vi "Phoenix.vi"() -> ()   [LabVIEW 2020]
uses:
  Vision_class/Old vision/SSL Detection Frame Simple Estimator Cameras VelCmd Folder/Core/AI Input.ctl
  Vision_class/Old vision/Controls/AI Robot.ctl
  Vision_class/Old vision/Controls/Functions Enum.ctl
  Vision_class/Old vision/Controls/AttackerStates.ctl
  Vision_class/Old vision/Controls/PathDests.ctl
  Vision_class/Old vision/Controls/PathDest.ctl
  Vision_class/Old vision/SSL Detection Frame Simple Estimator Cameras VelCmd Folder/Core/AI Ball.ctl
  Vision_class/Old vision/SSL Detection Frame Simple Estimator Cameras VelCmd Folder/Core/Field Size.ctl
  Vision_class/Old vision/SSL Detection Frame Simple Estimator Cameras VelCmd Folder/Core/AI Judge.ctl
  Communication_class/Paths/MessageAI_State Folder/Intel/Command Enum.ctl
  Vision_class/Old vision/SSL Detection Frame Simple Estimator Cameras VelCmd Folder/Util/Events/Events.ctl
  Vision_class/Old vision/Controls/Estimadores.ctl
  Vision_class/Old vision/Decode SSL and Refree Wrapper Package Folder/SSL Referee Game Status.ctl
  Vision_class/Old vision/Draw Field Folder/DrawTargets.ctl
  Vision_class/Old vision/Controls/SSL Field State.ctl
  Vision_class/Old vision/Controls/SSL Detection Frame.ctl
  Vision_class/Old vision/Controls/SSL Detection Robot.ctl
  <vilib>/Analysis/Matrix/Datatypes/RealMatrix.ctl
  Vision_class/Old vision/Controls/SSL Detection Ball.ctl
  Communication_class/Communication.lvclass
  Controls/ComUDP.ctl
  Controls/ComSerial.ctl
  Controls/ComSOS.ctl
  Controls/vision_control.ctl
  Team_class/KeeperPlay.ctl
  Team_class/OffensivePlay.ctl
  Referee_class/command_interpreted.ctl
  Robot_class/roles.ctl
  Robot_class/tactics.ctl
  Team_class/DefensivePlay.ctl
  Communication_class/Paths/grSim Packet Command UDP Test Folder/grSim/grSim RobotReplacement.ctl
  Communication_class/Paths/grSim Packet Command UDP Test Folder/grSim/grSim_BallReplacement.ctl
  Vision_class/Vision.lvclass
  Game_class/Game.lvclass
  Game_class/Game.lvclass/Game.ctl
  Parameters_class/Parameters.lvclass/Parameters.ctl
  Robot_class/Robot.lvclass
  Team_class/Team.lvclass/Team.ctl
  Events_class/Events.lvclass
  Referee_class/Referee.lvclass/Referee.ctl
  Robot_class/Robot.lvclass/Robot.ctl
  Game_class/Read KeeperTeam.vi
  Game_class/Write KeeperTeam.vi
  Game_class/Write Offensive ids.vi
  Game_class/Write Defensive ids.vi
  Game_class/Read Parameters.lvclass.vi
  Game_class/Write TestMode IDs.vi
  Game_class/Write TestMode.vi
  Game_class/Write Tests.vi
  Parameters_class/Write Area.vi
  Parameters_class/Write DistanceBehindAttacker.vi
  Parameters_class/Write DistanceInFrontOfAttacker.vi
  Parameters_class/Write DistanceStop.vi
  Parameters_class/Write DistanceToBallOut.vi
  Parameters_class/Write DistanceToGoAroundBall.vi
  Parameters_class/Write DistanceToGoAroundBallPass.vi
  Parameters_class/Write DistanceToKickingAngle.vi
  Parameters_class/Write Force++.vi
  Parameters_class/Write KickAngle.vi
  Parameters_class/Write KickEps.vi
  Parameters_class/Write KickForce.vi
  Parameters_class/Write KickRange.vi
  Parameters_class/Write MaxAcceleration.vi
  Parameters_class/Write MaxControlIncrement.vi
  Parameters_class/Write MaxDeceleration.vi
  Parameters_class/Write MaxOutputAngle.vi
  Parameters_class/Write MaxOutputXY.vi
  Parameters_class/Write MinDistToKick.vi
  Parameters_class/Write PassAngle.vi
  Parameters_class/Write Type of Marker.vi
  Parameters_class/Write AttackerFarback.vi
  Parameters_class/Write TouchDistance.vi
  Parameters_class/Write TimeoutDistanceInY.vi
  Parameters_class/Write TimeoutDistanceInX.vi
  Parameters_class/Write TimeoutDistanceBetweenRobots.vi
  Parameters_class/Write DistanceForPossession.vi
  Parameters_class/Write DistanceForaStillBall.vi
  Parameters_class/Write AngularToleranceForPossession.vi
  Parameters_class/Write AttakingOurselves.vi
  Parameters_class/Write Debug.vi
  Parameters_class/Write ChipKick activated.vi
  Parameters_class/Write Angle.vi
  Parameters_class/Write PID gains Vel.vi
  Parameters_class/Write PID gains Vel_desired.vi
  Parameters_class/Write PID gains Angle.vi
  Parameters_class/Write Number of Offesnive.vi
  Parameters_class/Write Shoot Out_.vi
  Parameters_class/Write DefenseAvoidArea.vi
  Parameters_class/Write InvertKick.vi
  Game_class/Write Parameters.lvclass.vi
  Game_class/Read DefensiveTeam.vi
  Team_class/Read RobotRef.vi
  Game_class/Read OffensiveTeam.vi
  Game_class/Read AllyRef.vi
  Team_class/Write RobotRef.vi
  Game_class/Write NavigationTeam.vi
  Game_class/Write EventsRef.vi
  Game_class/Write OffensiveTeam.vi
  Robot_class/Read id.vi
  Robot_class/Read role.vi
  Robot_class/Read tactic.vi
  Game_class/Read Referee.vi
  Team_class/Read DefensivePlay.vi
  Team_class/Read OffensivePlay.vi
  Team_class/Read KeeperPlay.vi
  Referee_class/Read command_interpreted.vi
  Game_class/Read EventsRef.vi
  Ally_class/Ally.lvclass
  Playbook_class/Playbook.lvclass
  Parameters_class/Parameters.lvclass
  Referee_class/Referee.lvclass
  Utilities_class/Utilities.lvclass
  <vilib>/Analysis/Matrix/NI_Matrix.lvlib
panel:
  out "FPS vision 2":dbl
  out "FPS Offensive 2":dbl
  in  "grSIM replacement":cluster{"robots":T1[], "ball":T2}
  in  "replace active":bool
  out "Vel estimativa":T3(graph)
  out "Vel cmd":T3(graph)
  in  "Debug":bool
  out "tempo udp":dbl
  in  "ball out":bool
  in  "ball velocity máx":dbl=20.0
  in  "PID gains Angle":cluster{"(Kc)":dbl, "(Ki)":dbl, "(Kd)":dbl}={"(Kc)"=5.0, "(Ki)"=0.1, "(Kd)"=-1.0}
  in  "PID gains Vel D":cluster{"(Kp)":dbl, "(Ki)":dbl, "(Kd)":dbl}={"(Kp)"=20.0, "(Ki)"=100.0, "(Kd)"=0.5}
  in  "ChipKick activated":bool
  out "error out":errorcluster
  in  "Draw Graphs":bool
  out "zoom":dbl
  in  "Test":bool
  in  "Tab Control":T4(tab)
  in  "Com UDP":T5={"UDP GrSim TX"=TRUE, "Address:"="127.0.0.1", "Port:"=20011}
  in  "Com Serial":T6={"Serial TX"=FALSE, "Porta:"="COM12"}
  in  "Com SOS":T7={"UDP SOS TX "=FALSE, "SOS Port: 2"=10025, "SOS Port: "=10021, "SOS Address:"="192.168.0.101"}
  in  "RefBox UDP RX":T8={"Local IP:"="", "Port"=10003, "Server IP:"="224.5.23.1"}
  out "RefBox RX":bool
  in  "Defense\n stretch":i32=2000
  in  "Defense\n width":i32=1000
  in  "Team":enum16{"Azul", "Amarelo"}(ring) caption="Enum"
  in  "Side":enum16{"Esquerdo", "Direito"}(ring) caption="Enum"
  in  "Goalie":string(combo)="0"
  in  "Command":string(combo)="Auto"
  in  "AttakingOurselves":bool
  out "SSL RX":bool
  in  "SSL UDP RX":T8={"Local IP:"="", "Port"=10020, "Server IP:"="224.5.23.2"}
  out "KeeperPlay":T9=enum."NormalGame"
  out "OffensivePlay":T10=enum."TestPlay"
  out "Keeper Team":cluster{"id":i32, "role":T11, "tactic":T12}[](array[cluster])
  out "Offensive Team":cluster{"id":i32, "role":T11, "tactic":T12}[](array[cluster])
  out "Defensive Team":cluster{"id":i32, "role":T11, "tactic":T12}[](array[cluster])
  out "DefensivePlay":T13=enum."Halt"
  in  "TestMode IDS":dbl[](array[numeric])
  out "SSL Referee Game Status":T14 {"Time" format="%<%.3X %x>T"; "Blue Timeout Remaining" format="%<%M:%S>t"; "Yellow Timeout Remaining" format="%<%M:%S>t"; "Time Left" format="%<%M:%S>t"}
  out "FPS Offensive":dbl
  out "FPS SetParameters":dbl
  out "FPS Com":dbl
  out "FPS Draw Field":dbl
  out "FPS Graph":dbl
  out "FPS referee":dbl
  out "FPS vision":dbl
  out "FPS Events":dbl
  out "FPS Mouse":dbl
  out "FPS Print Field":dbl
  in  "zigzag Points":cluster{"x":dbl, "y":dbl, "Angle":dbl}[](array[cluster])=[{"x"=-4300.0, "y"=-3000.0, "Angle"=0.0}, {"x"=-4300.0, "y"=3000.0, "Angle"=0.0}, {"x"=-100.0, "y"=3000.0, "Angle"=0.0}, {"x"=-4300.0, "y"=3000.0, "Angle"=0.0}]
  in  "TestMode":bool
  in  "Tests":enum16{"zigzag", "goto"}(ring)
  in  "Offensive ids":dbl[](array[numeric])
  in  "Defensive ids":dbl[](array[numeric])
  out "command_interpreted":T15=enum."Halt"
  out "FPS Navigation":dbl
  out "FPS Read UDP":dbl
  in  "id 3":dbl
  in  "id 2":dbl
  in  "id 1":dbl
  out "Robot":cluster{"Modulo":dbl, "Modulo":dbl}(graph)
  out "Robot":cluster{"Modulo":dbl, "Modulo":dbl}(graph)
  out "Robot":cluster{"Modulo":dbl, "Modulo":dbl}(graph)
  out "ball":dbl(graph)
  in  "AI Parameters":T16={"Defensive Marker"=enum."SecondMostDangerous", "TimeoutDistanceInX"=600.0, "TimeoutDistanceInY"=600.0, "DistanceForaStillBall"=0.0, "TouchDistance"=130.0, "AttackerFarback"=1500.0, "MinDistToKick"=150.0, "Type of Marker"=enum."BlockEnemyPass", "Type of Defense "=enum."Manmark", "PassAngle"=0.045, "KickRange"=60.0, "KickForce"=100.0, "KickEps"=0.05, "KickAngle"=0.09, "Force++"=5.0, "DistanceToKickingAngle"=150.0, "DistanceToBallOut"=600.0, "DistanceStop"=600.0, "DistanceBehindAttacker"=200.0, "Area"=enum."Square", "DistanceForPossession"=180.0, "DistanceToGoAroundBallPass"=0.0, "DistanceToGoAroundBall"=200.0, "DistanceInFrontOfAttacker"=200.0, "TimeoutDistanceBetweenRobots"=300.0, "MaxOutputAngle"=4.0, "MaxOutputXY"=1.0, "MaxDeceleration"=1.0, "MaxControlIncrement"=1.0, "MaxAcceleration"=4.0, "AngularToleranceForPossession"=0.3, "MaxVelBallToBeginDuelist"=0.5, "ZigZagAngle"=0.0, "PID gains Vel"={"(Kc)"=0.0, "(Ti, min)"=0.0, "(Td, min)"=0.0}, "Number of Offensive"=enum."Auto", "Shoot Out?"=FALSE, "DefenseAvoidArea"=FALSE, "InvertKick"=[]}
  in  "Id camera\ninf dir":dbl=2.0
  in  "Id camera\ninf esq":dbl
  in  "Id camera\nsup dir":dbl=3.0
  in  "Id camera\nsup esq":dbl=1.0
  in  "ignore left?":bool
  in  "ignore rigth?":bool
  in  "Estimador":T17=enum."Kalman"
  in  "Draw Targets?":T18={"Attacker"=TRUE, "Striker"=TRUE, "Goalie"=TRUE, "Defender"=TRUE, "kick"=TRUE, "Est Ball"=TRUE, "Est Robot"=FALSE, "Path S"=FALSE, "Path C"=FALSE, "Dngr.Enemy"=TRUE, "2nd Striker"=TRUE}
  in  "Draw Field":bool=TRUE
  in  "Communication in":refnum<class "Communication.lvclass">
  in  "Frame and Field Size out Ref":T19 {"Detection Frame Out"."robots_blue"."height" format="%+4.3f"; "Detection Frame Out"."robots_blue"."pixel_y" format="%+4.3f"; "Detection Frame Out"."robots_blue"."pixel_x" format="%+4.3f"; "Detection Frame Out"."robots_blue"."orientation" format="%+4.3f"; "Detection Frame Out"."robots_blue"."y" format="%+4.3f"; "Detection Frame Out"."robots_blue"."confidence" format="%4.3f"; "Detection Frame Out"."robots_blue"."x" format="%+4.3f"; "Detection Frame Out"."robots_yellow"."height" format="%+4.3f"; "Detection Frame Out"."robots_yellow"."pixel_y" format="%+4.3f"; "Detection Frame Out"."robots_yellow"."pixel_x" format="%+4.3f"; "Detection Frame Out"."robots_yellow"."orientation" format="%+4.3f"; "Detection Frame Out"."robots_yellow"."y" format="%+4.3f"; "Detection Frame Out"."robots_yellow"."confidence" format="%4.3f"; "Detection Frame Out"."robots_yellow"."x" format="%+4.3f"}
  out "2D Picture":picture
  in  "SSL Referee Game Status Ref":T14 {"Time" format="%<%.3X %x>T"; "Blue Timeout Remaining" format="%<%M:%S>t"; "Yellow Timeout Remaining" format="%<%M:%S>t"; "Time Left" format="%<%M:%S>t"}
  out "GUI Game Status":T14 {"Time" format="%<%.3X %x>T"; "Blue Timeout Remaining" format="%<%M:%S>t"; "Yellow Timeout Remaining" format="%<%M:%S>t"; "Time Left" format="%<%M:%S>t"}
  out "AI State":T24={"our_robots"=[], "enemy_robots"=[], "balls"=[], "geometry"={"line_width"=0, "field_length"=0, "field_width"=0, "boundary_width"=0, "referee_width"=0, "goal_width"=0, "goal_depth"=0, "goal_wall_width"=0, "center_circle_radius"=0, "defense_radius"=0, "defense_stretch"=0, "free_kick_from_defense_dist"=0, "penalty_spot_from_field_line_dist"=0, "penalty_line_from_spot_dist"=0}, "IA Judge"={"stage"="", "command"="", "our_goalie_id"=0.0, "enemy_goalie_id"=0.0, "command enum"=enum."Halt", "Time"=enum."Azul"}, "Received Timestamp"=timestamp(0 s since 1904-01-01), "Events"={"Touch"=FALSE, "Ball out"=FALSE, "id touch"=0.0, "Ball out of \nVision"=FALSE, "Ball inside \nGoalie area"=FALSE, "Robot not responding"=FALSE, "Robots responding status"=[1.0, 1.0, 1.0, 1.0, 1.0, 1.0], "Enemy Ball \nPossession"=FALSE, "Pass State"=FALSE, "id end of pass"=0.0, "Kick"=FALSE, "Id ini Possession"=0.0, "Ball Possesion"=FALSE, "Id Possesion"=0.0, "Direct Kick"=FALSE, "2nd Strk Ativo"=FALSE}}
  # "To execute Test and TestMode(zigzag)\nthe referee command must be Stop"
  # "PID gains vel:\nmakes the estimated velocity\ngoes closer into the desired velocity"
  # "Score"
  # "Red Cards"
  # "Yellow Cards"
  # "Timeouts Left"
  # "Timeout Remaining"
  # "Goalie ID"
  # "left goal"
  # "right goal"
  # "vision computer"
  # "Score"
  # "Red Cards"
  # "Yellow Cards"
  # "Timeouts Left"
  # "Timeout Remaining"
  # "Goalie ID"
  # "Score"
  # "Red Cards"
  # "Yellow Cards"
  # "Timeouts Left"
  # "Timeout Remaining"
  # "Goalie ID"
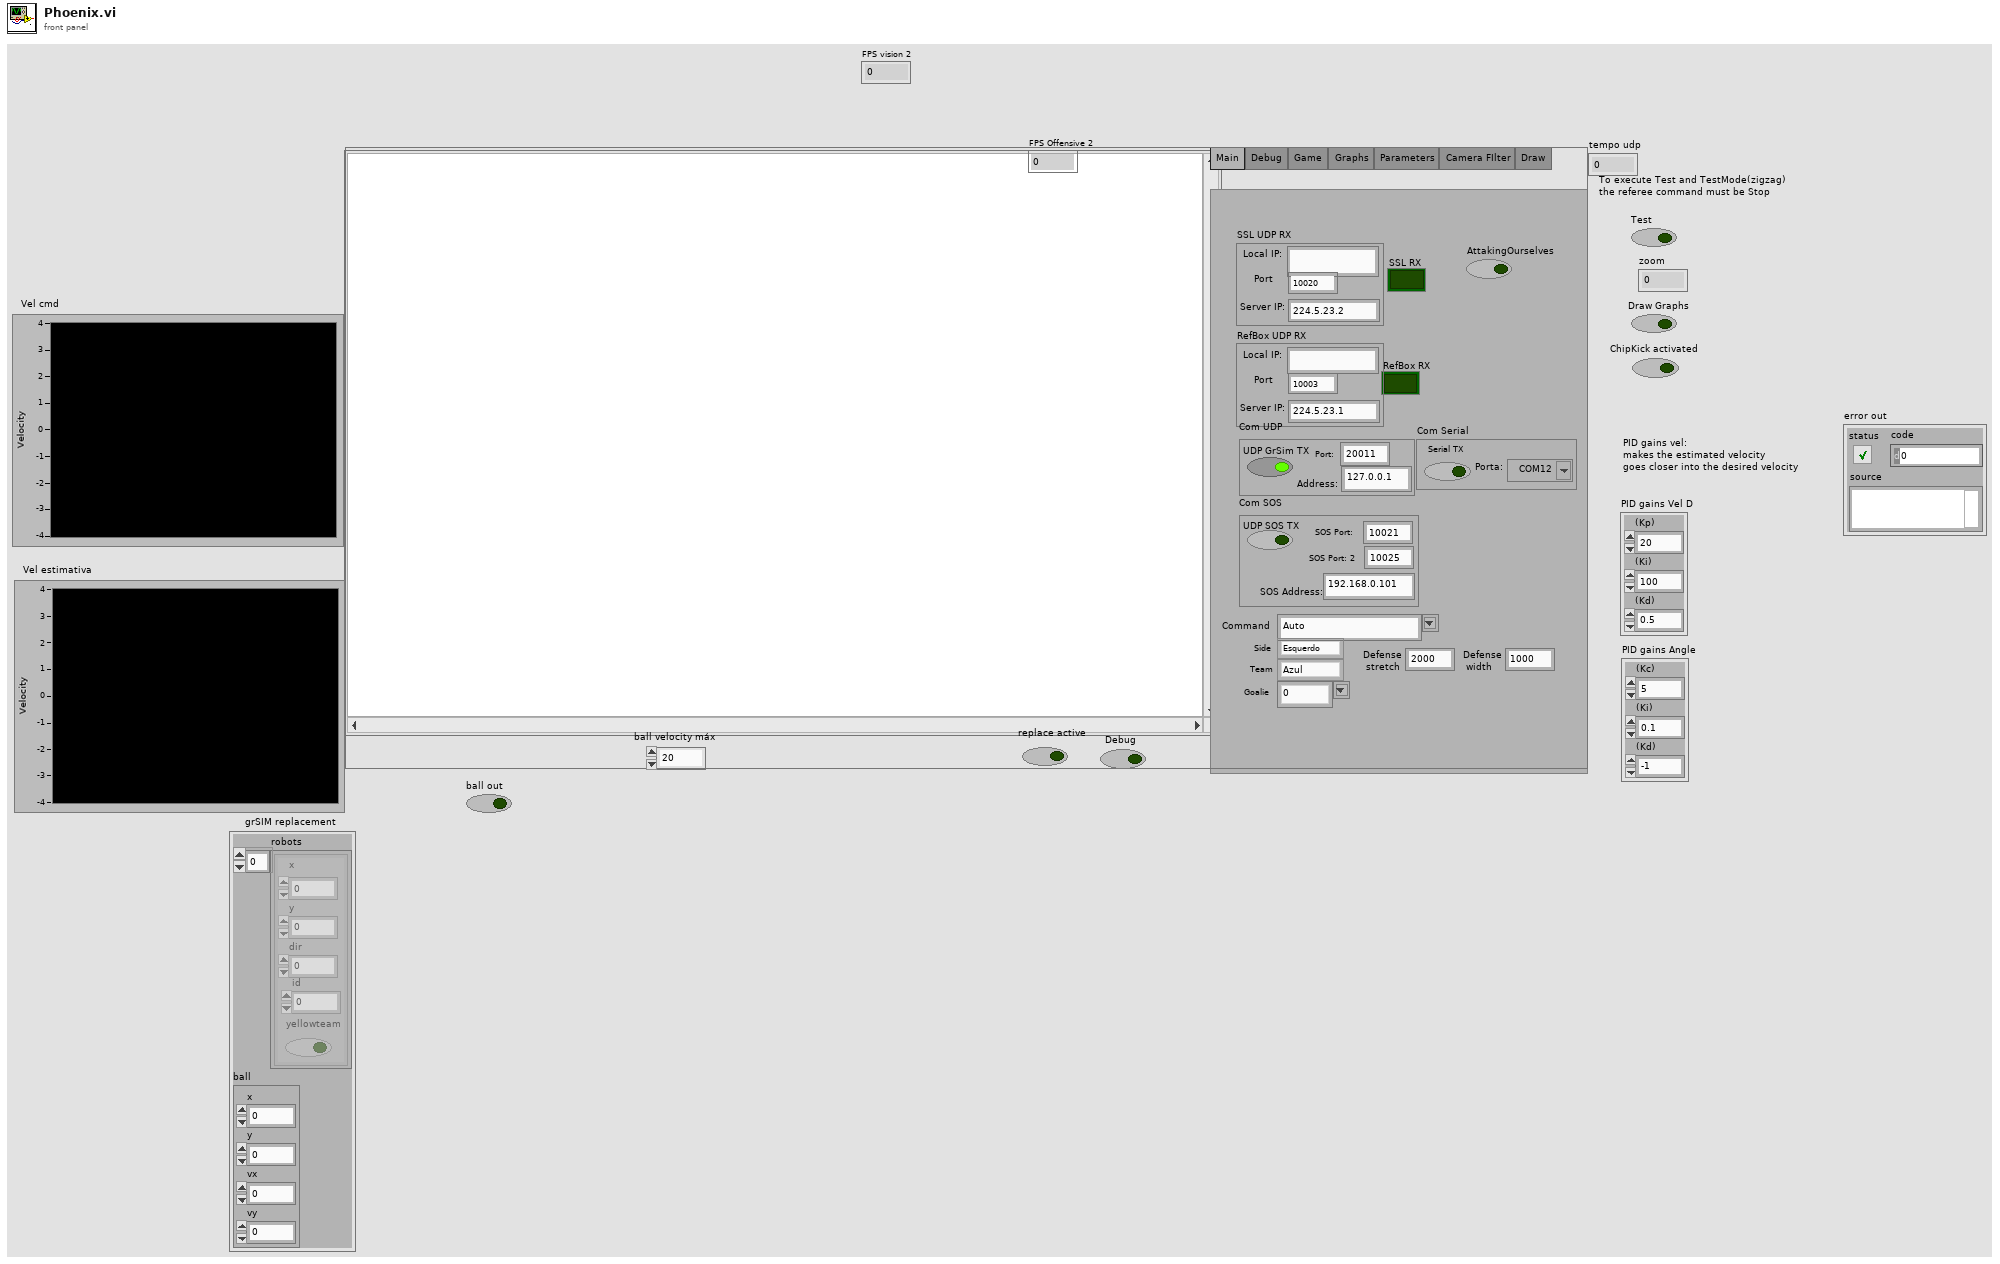
[diagram p1: front panel]
types:
  T1 = typedef "grSim RobotReplacement.ctl" = cluster{"x":dbl, "y":dbl, "dir":dbl, "yellowteam":bool, "id":u32}
  T2 = typedef "grSim_BallReplacement.ctl" = cluster{"x":dbl, "y":dbl, "vx":dbl, "vy":dbl}
  T3 = cluster{"v_norm":dbl, "v_tang":dbl, "Modulo":dbl}
  T4 = enum32{"Main", "Debug", "Game", "Graphs", "Parameters", "Camera FIlter", "Draw"}
  T5 = typedef "ComUDP.ctl" = cluster{"UDP GrSim TX":bool, "Address:":string, "Port:":u16}
  T6 = typedef "ComSerial.ctl" = cluster{"Serial TX":bool, "Porta:":refnum<visa-resource-name>}
  T7 = typedef "ComSOS.ctl" = cluster{"UDP SOS TX ":bool, "SOS Port: 2":u16, "SOS Port: ":u16, "SOS Address:":string}
  T8 = typedef "vision_control.ctl" = cluster{"Local IP:":string, "Port":i32, "Server IP:":string}
  T9 = typedef "KeeperPlay.ctl" = enum16{"ZigZag", "Goto", "NormalGame", "KeeperPlay", "Halt", "Timeout", "PenaltyEnemy", "TestPlay"}
  T10 = typedef "OffensivePlay.ctl" = enum16{"PreparePass", "PassToStriker", "BallOutOfField", "PassTo2ndStriker", "StopOffensive", "Prepare Penalty Enemy", "EnemyPossessionAtEnemyField", "EnemyPossesionAtOurField", "TestPlay", "PreparePenaltyAlly", "KickPenaltyAlly", "PrepareKickoffAlly", "PrepareKickoffEnemy", "IndirectEnemy", "DirectEnemy", "NormalGame", "DirectKick", "Pass", "Halt", "Timeout", "PassPlay", "PenaltyEnemy"}
  T11 = typedef "roles.ctl" = enum16{"PenaltyDefense", "DefaultPs", "PreparePassReceiver", "PassObserver", "Timeout", "Goto", "ZigZag", "None", "BallOutOfField", "DefenderArea", "Duelist", "AttackerStop", "FollowAttacker", "KeeperRole", "KickPenalty", "AttackerAimGoal", "AttackerBlock", "Marker", "Halt", "Shoot", "PassKicker", "PassReceiver", "TestRole", "PenaltyAttacker"}
  T12 = typedef "tactics.ctl" = enum16{"PenaltyAttacker", "DefaultPs", "PassObserver", "PenaltyDefense", "Test", "DefendGoal", "Marker", "FollowAttacker", "DefendArea", "Shoot", "AttackerAimGoal", "AttackerBallOutOfField", "AttackerBlock", "AttackerStop", "Duelist", "Halt", "ZigZag", "GoTo", "Timeout", "KickToPassReceiver", "PositionToReceivePass", "PassReceiver", "WaitPass"}
  T13 = typedef "DefensivePlay.ctl" = enum16{"NormalDefensiveWithDuelist", "NormalDefensive", "TestPlay", "Halt", "Timeout", "PenaltyEnemy", "PenaltyAlly"}
  T14 = typedef "SSL Referee Game Status.ctl" = cluster{"Stage":string, "Command":string, "Time Left":dbl, "Yellow Team":string, "Blue Team":string, "Yellow Score":u32, "Blue Score":u32, "Yellow Red Cards":u32, "Blue Red Cards":u32, "Yellow Yellow Cards":u32, "Blue Yellow Cards":u32, "Yellow Timeouts Left":u32, "Blue Timeouts Left":u32, "Yellow Timeout Remaining":dbl, "Blue Timeout Remaining":dbl, "Yellow Goalie Id":u32, "Blue Goalie Id":u32, "Time":timestamp}
  T15 = typedef "command_interpreted.ctl" = enum16{"Goal Ally", "Goal Enemy", "Ball Placement Enemy", "Ball Placement Ally", "Normal Half Time", "Extra Time  Break", "Extra Half Time", "None", "Post Game", "PKA Normal Start", "Prepare Kickoff Ally", "PKE Normal Start", "Prepare Kickoff Enemy", "Force Start", "Halt", "Timeout", "Prepare Penalty Ally", "Prepare Penalty Enemy", "PPA NormalStart", "PPE Normal Start", "Indirect Free Ally", "Direct Free Enemy", "Direct Free Ally", "Indirect Free Enemy", "Stop"}
  T16 = cluster{"Defensive Marker":enum16{"SecondMostDangerous", "MostDangerous"}, "TimeoutDistanceInX":dbl, "TimeoutDistanceInY":dbl, "DistanceForaStillBall":dbl, "TouchDistance":dbl, "AttackerFarback":dbl, "MinDistToKick":dbl, "Type of Marker":enum16{"BlockEnemyPass", "BlockOurGoal"}, "Type of Defense ":enum16{"Barreira", "Manmark"}, "PassAngle":dbl, "KickRange":dbl, "KickForce":dbl, "KickEps":dbl, "KickAngle":dbl, "Force++":dbl, "DistanceToKickingAngle":dbl, "DistanceToBallOut":dbl, "DistanceStop":dbl, "DistanceBehindAttacker":dbl, "Area":enum16{"Circular", "Square"}, "DistanceForPossession":dbl, "DistanceToGoAroundBallPass":dbl, "DistanceToGoAroundBall":dbl, "DistanceInFrontOfAttacker":dbl, "TimeoutDistanceBetweenRobots":dbl, "MaxOutputAngle":dbl, "MaxOutputXY":dbl, "MaxDeceleration":dbl, "MaxControlIncrement":dbl, "MaxAcceleration":dbl, "AngularToleranceForPossession":dbl, "MaxVelBallToBeginDuelist":dbl, "ZigZagAngle":dbl, "PID gains Vel":cluster{"(Kc)":dbl, "(Ti, min)":dbl, "(Td, min)":dbl}, "Number of Offensive":enum16{"6", "5", "4", "3", "2", "1", "0", "Auto"}, "Shoot Out?":bool, "DefenseAvoidArea":bool, "InvertKick":dbl[]}
  T17 = typedef "Estimadores.ctl" = enum16{"Nenhum", "Simples", "Kalman"}
  T18 = typedef "DrawTargets.ctl" = cluster{"Attacker":bool, "Striker":bool, "Goalie":bool, "Defender":bool, "kick":bool, "Est Ball":bool, "Est Robot":bool, "Path S":bool, "Path C":bool, "Dngr.Enemy":bool, "2nd Striker":bool}
  T19 = typedef "SSL Field State.ctl" = cluster{"Detection Frame Out":T20, "Field Size Out":cluster{"line_width":u32, "field_length":u32, "field_width":u32, "boundary_width":u32, "referee_width":u32, "goal_width":u32, "goal_depth":u32, "goal_wall_width":u32, "center_circle_radius":u32, "defense_radius":u32, "defense_stretch":u32, "free_kick_from_defense_dist":u32, "penalty_spot_from_field_line_dist":u32, "penalty_line_from_spot_dist":u32}, "Received Time Stamp":timestamp}
  T20 = typedef "SSL Detection Frame.ctl" = cluster{"frame_number":u32, "t_capture":dbl, "t_sent":dbl, "camera_id":u32, "robots_yellow":T21[], "robots_blue":T21[], "balls":T23[], "Valid":bool, "Time Stamp":timestamp}
  T21 = typedef "SSL Detection Robot.ctl" = cluster{"x":sgl, "robot_id":u32, "confidence":sgl, "y":sgl, "orientation":sgl, "pixel_x":sgl, "pixel_y":sgl, "height":sgl, "Valid":bool, "Time Stamp":timestamp, "x_k|k":T22, "Pk|k":T22, "Previous Time Stamp":timestamp, "R":T22}
  T22 = typedef "NI_Matrix.lvlib/RealMatrix.ctl" = dbl[][]
  T23 = typedef "SSL Detection Ball.ctl" = cluster{"x":sgl, "area":u32, "confidence":sgl, "y":sgl, "z":sgl, "pixel_x":sgl, "pixel_y":sgl, "Valid":bool, "Time Stamp":timestamp, "x_k|k":T22, "Pk|k":T22, "Id":u32, "Previous Time Stamp":timestamp, "R":T22}
  T24 = typedef "AI Input.ctl" = cluster{"our_robots":T25[], "enemy_robots":T25[], "balls":T30[], "geometry":T31, "IA Judge":T32, "Received Timestamp":timestamp, "Events":T34}
  T25 = typedef "AI Robot.ctl" = cluster{"id":u32, "function":T26, "x":dbl, "y":dbl, "orientation":dbl, "v_tangent":dbl, "v_normal":dbl, "v_ang":dbl, "kick_x":dbl, "kick_z":dbl, "dribble":bool, "Timestamp":timestamp, "estimatives":cluster{"est_v_tangent":dbl, "est_v_normal":dbl, "est_vx":dbl, "est_vy":dbl, "Pos Robot Est":dbl[]}, "dest_x_kick":dbl, "dest_y_kick":dbl, "Gap Coord":dbl[], "States":T27, "Path ":dbl[][], "Path  Smooth":dbl[][], "Dest":T28, "vx_desired":dbl, "vy_desired":dbl}
  T26 = typedef "Functions Enum.ctl" = enum16{"2nd Striker", "Attacker", "Goalie", "Defender", "Striker", "Goto 0", "Dummy", "Kicker", "ZigZag 0", "ZigZag 1", "ZigZag 2", "ZigZag 3", "ZigZag 4", "ZigZag 5", "ZigZag 6", "ZigZag 7", "ZigZag 8", ""}
  T27 = typedef "AttackerStates.ctl" = enum16{"Pass", "GoToTangent", "BallGetting", "GoToKick", ""}
  T28 = typedef "PathDests.ctl" = T29[]
  T29 = typedef "PathDest.ctl" = cluster{"dest_x":dbl, "dest_y":dbl, "dest_orientation":dbl, "dest_vel":dbl}
  T30 = typedef "AI Ball.ctl" = cluster{"x":dbl, "y":dbl, "timestamp":timestamp, "Vel_x":dbl, "Vel_y":dbl, "Pos Bola Est":dbl[], "Valid":bool}
  T31 = typedef "Field Size.ctl" = cluster{"line_width":u32, "field_length":u32, "field_width":u32, "boundary_width":u32, "referee_width":u32, "goal_width":u32, "goal_depth":u32, "goal_wall_width":u32, "center_circle_radius":u32, "defense_radius":u32, "defense_stretch":u32, "free_kick_from_defense_dist":u32, "penalty_spot_from_field_line_dist":u32, "penalty_line_from_spot_dist":u32}
  T32 = typedef "AI Judge.ctl" = cluster{"stage":string, "command":string, "our_goalie_id":dbl, "enemy_goalie_id":dbl, "command enum":T33, "Time":enum16{"Azul", "Amarelo"}}
  T33 = typedef "Command Enum.ctl" = enum16{"Halt", "Stop", "Force Start", "PKA Normal Start", "Prepare Kickoff Ally", "PKE Normal Start", "Prepare Kickoff Enemy", "Prepare Penalty Ally", "PPA Normal Start", "Prepare Penalty Enemy", "PPE Normal Start", "Direct Free Enemy", "Direct Free Ally", "Indirect Free Enemy", "Indirect Free Ally", "Timeout Enemy", "Timeout Ally", "Goal Enemy", "Goal Ally", "Ball Placement Enemy", "Ball Placement Ally", "Normal Half Time", "Extra Time Break", "Extra Half Time", "None", "Post Game"}
  T34 = typedef "Events.ctl" = cluster{"Touch":bool, "Ball out":bool, "id touch":dbl, "Ball out of \nVision":bool, "Ball inside \nGoalie area":bool, "Robot not responding":bool, "Robots responding status":dbl[], "Enemy Ball \nPossession":bool, "Pass State":bool, "id end of pass":dbl, "Kick":bool, "Id ini Possession":dbl, "Ball Possesion":bool, "Id Possesion":dbl, "Direct Kick":bool, "2nd Strk Ativo":bool}
  T35 = cluster{"(Kc)":dbl, "(Ti, min)":dbl, "(Td, min)":dbl}
  T36 = enum16{"6", "5", "4", "3", "2", "1", "0", "Auto"}
  T37 = cluster{"est_v_norm":dbl, "est_v_tang":dbl, "Modulo":dbl}
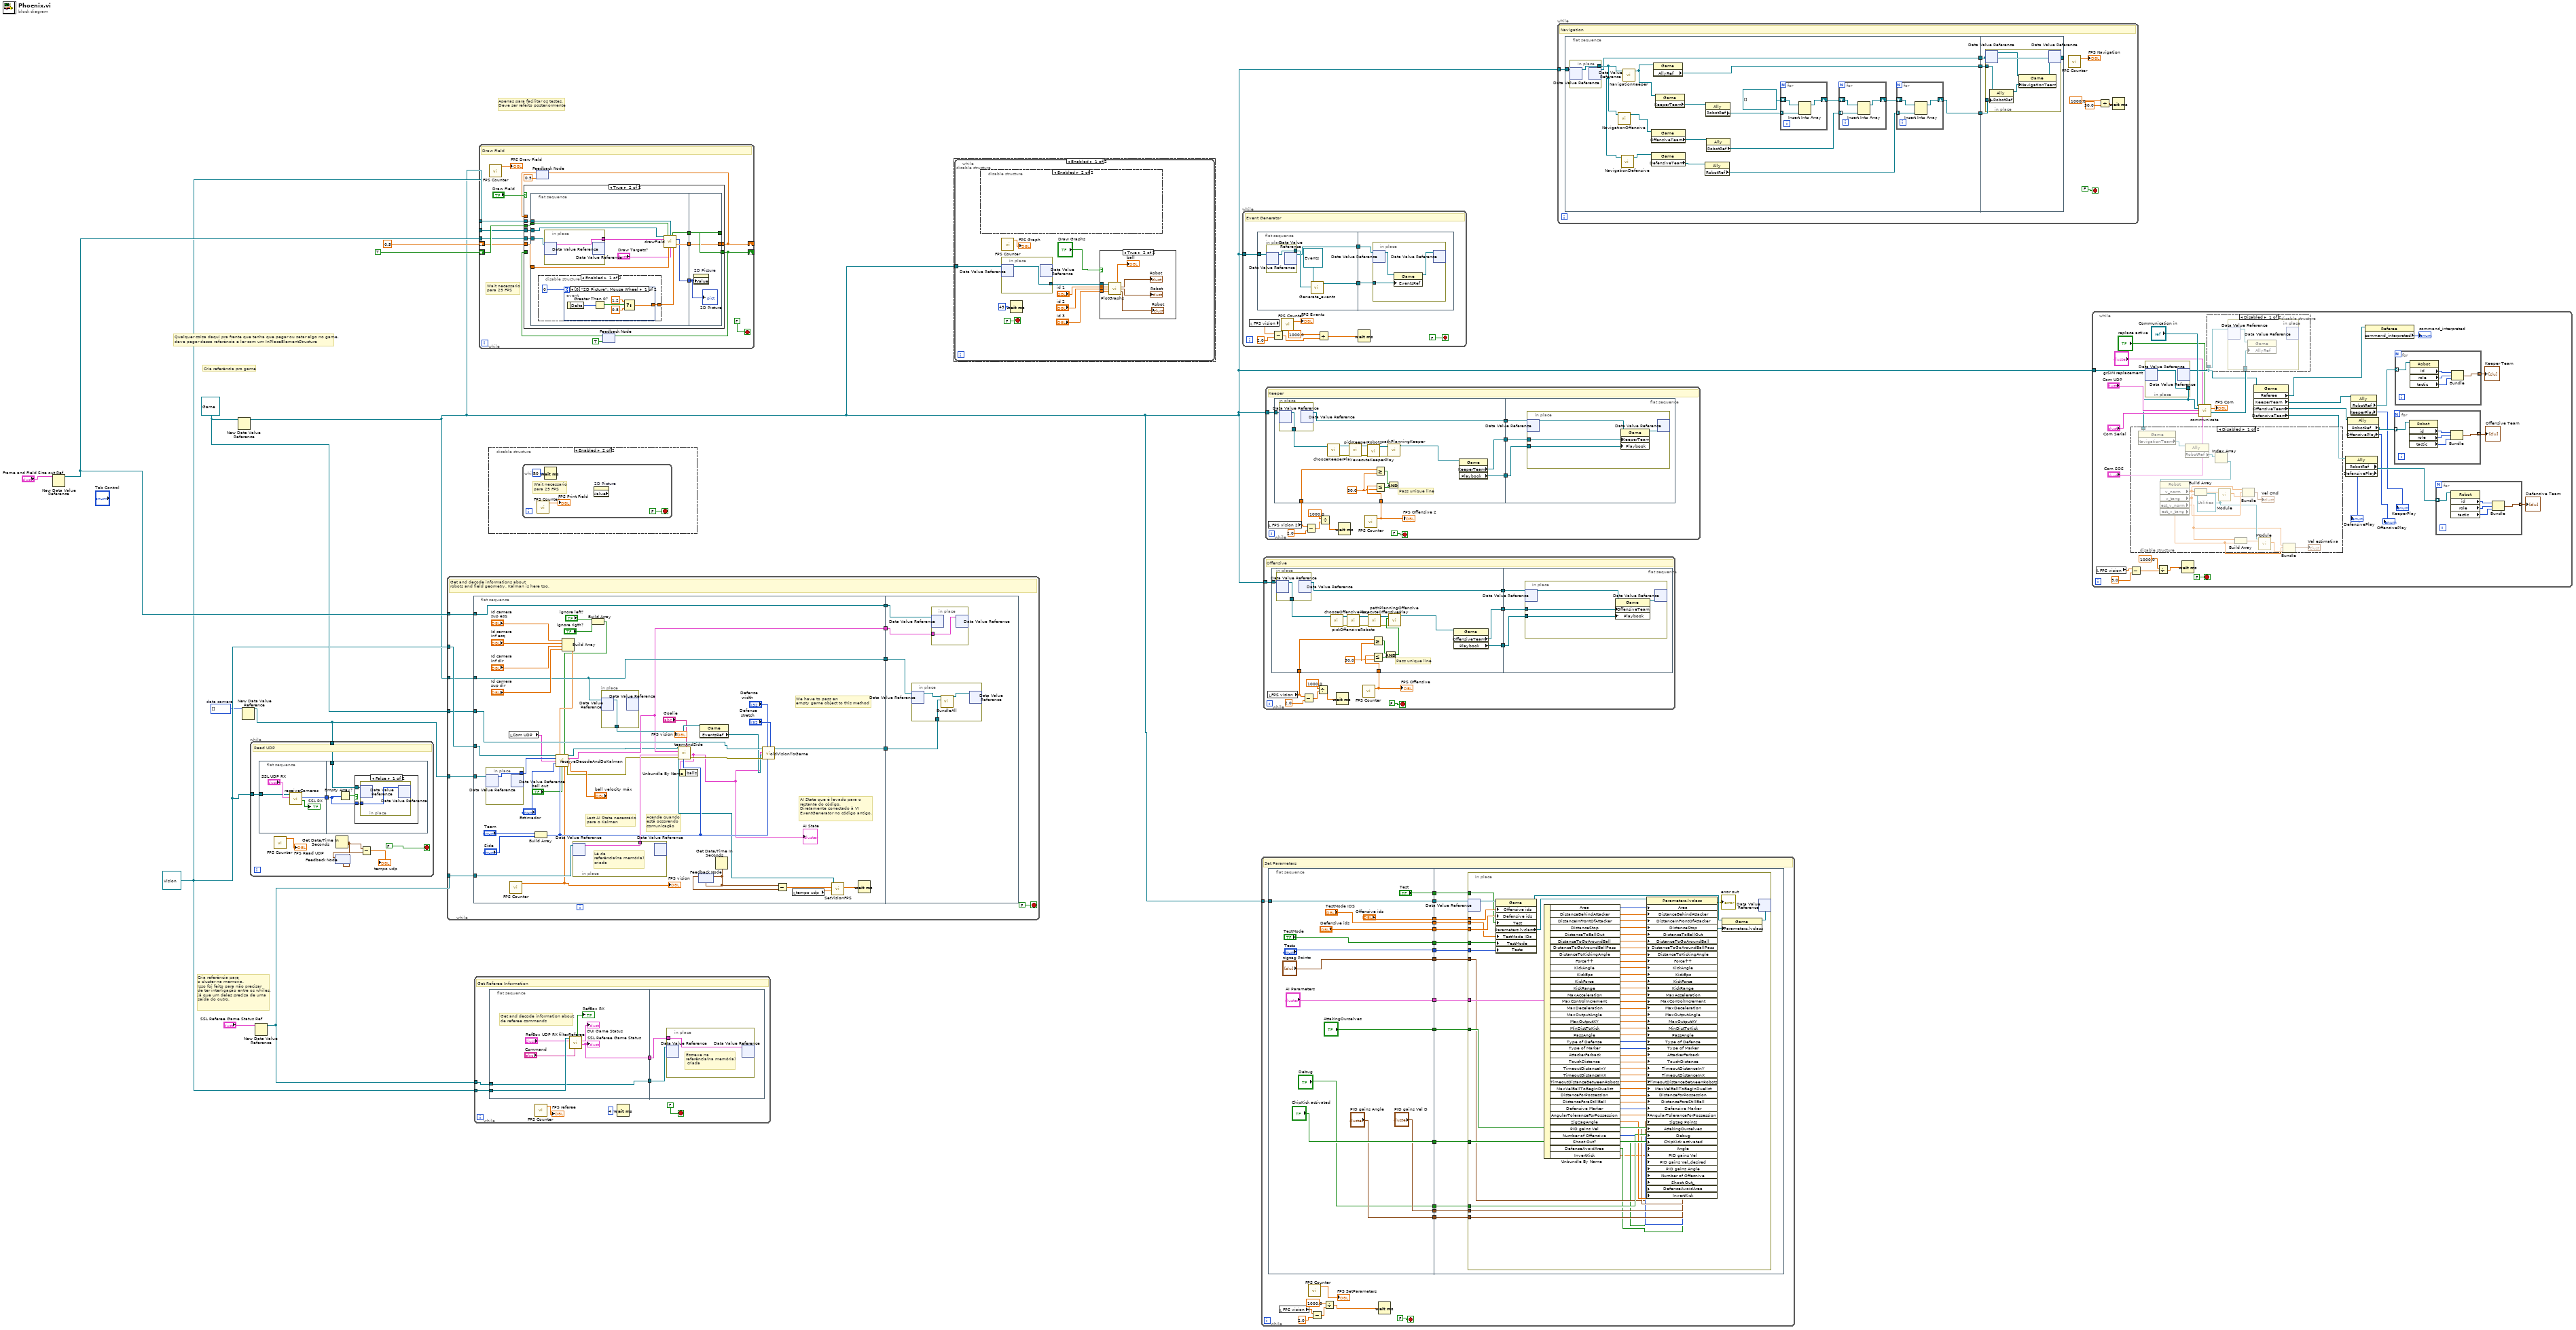
[diagram p0: block diagram]
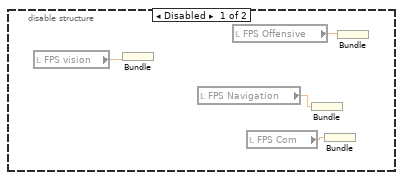
[diagram p3: hidden frame]
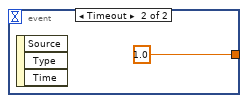
[diagram p7: hidden frame]
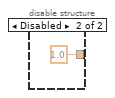
[diagram p8: hidden frame]
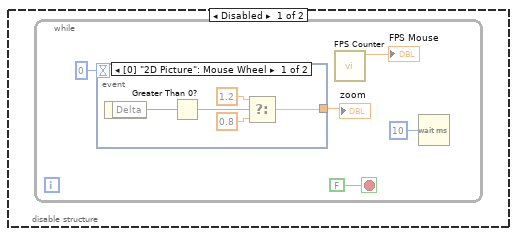
[diagram p9: hidden frame]
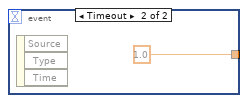
[diagram p10: hidden frame]
diagram:
  w3 = u8[] []  # data camera
  w5 = refnum<class "Game.lvclass"> refnum ("Game")
  w4 = refnum<class "Vision.lvclass"> refnum ("Vision")
  # "Apenas para facilitar os testes.\nDeve ser refeito posteriormente"
  # "Qualquer coisa daqui pra frente que tenha que pegar ou setar algo no game,\ndeve pegar dessa referência e ler com um InPlaceElementStructure"
  # "Cria referência pro game"
  # "Cria referência para\no cluster na memória.\nIsso foi feito para não precisar\nde ter interligação entre os whiles,\njá que um deles precisa de uma\nsaída do outro."
  n1 = New Data Value Reference(data value="Frame and Field Size out Ref") -> (data value reference=w6:refnum<data-value>)  [unwired: 1 in, 1 out]
  n2 = New Data Value Reference(data value=w5) -> (data value reference=w1:refnum<data-value>)  [unwired: 1 in, 1 out]
  n3 = New Data Value Reference(data value=w3) -> (data value reference=w2:refnum<data-value>)  [unwired: 1 in, 1 out]
  n4 = while {
    tunnel: w4 -> [w18]
    tunnel: w2 -> [w17]
    stop <- FALSE stop-if-true
    # "Read UDP"
    n5 = flat-sequence {
      tunnel: w18 -> [w22]
      tunnel: [w20] -> w16
      tunnel: w17 -> [w26]
      tunnel: w16 -> [w25]
      frame #0 {
        n6 = call "receiveCameras.vi"("Cluster"="SSL UDP RX", "Vision in"=w22) -> ("RX"=→"SSL RX":bool, "data camera out"=w20:u8[])  [unwired: 5 in, 2 out]
      }
      frame #1 {
        n7 = Empty Array?(array=w25) -> (empty?=w24:bool)
        n8 = case shown="False" w24 {
          tunnel: w26 -> [w28 _]
          tunnel: w25 -> [w27 _]
          frame False {
            n9 = in-place {
              in-place-border: w27 -> [w29]
              n10 = in-place-dvr #1(w28) -> ()  [unwired: 2 out]
              n11 = in-place-dvr #1(w29) -> ()  [unwired: 2 out]
            }
          }
          frame True {
          }
        }
      }
    }
    n12 = call "FPS Counter.vi"() -> ("Numeric"=→"FPS Read UDP":dbl)  [unwired: 11 in]
    n13 = Get Date/Time In Seconds() -> (seconds since 1Jan1904=w13:timestamp)
    n14 = feedback #2(w13) -> (w14:timestamp)
    n15 = feedback-in #2(w13) -> ()
    n16 = Subtract(x=w13, y=w14) -> (x-y=→"tempo udp":dbl)
  }
  n17 = New Data Value Reference(data value="SSL Referee Game Status Ref") -> (data value reference=w10:refnum<data-value>)  [unwired: 1 in, 1 out]
  n18 = while {
    tunnel: w4 -> [w39]
    tunnel: w10 -> [w38]
    tunnel: w1 -> [w35]
    tunnel: w6 -> [w36]
    tunnel: w5 -> [w37]
    tunnel: w2 -> [w30]
    stop <- FALSE stop-if-true
    # "Get and decode informations about\nrobots and field geometry. Kalman is here too."
    n19 = flat-sequence {
      tunnel: w39 -> [w55]
      tunnel: w38 -> [w79]
      tunnel: w37 -> [w64]
      tunnel: w36 -> [w66]
      tunnel: w35 -> [w65]
      tunnel: [w78] -> w34
      tunnel: [w53] -> w33
      tunnel: [w66] -> w32
      tunnel: [w65] -> w31
      tunnel: w30 -> [w60]
      tunnel: w34 -> [w86]
      tunnel: w33 -> [w84]
      tunnel: w32 -> [w85]
      tunnel: w31 -> [w87]
      frame #0 {
        # "We have to pass an\nempty game object to this method"
        # "Acende quando\nestá occorendo\ncomunicação"
        # "Last AI State necessário\npara o Kalman"
        # "AI State que é levado para o\nrestante do código.\nDiretamente conectado à VI\nEventGenerator no código antigo."
        n20 = in-place {
          in-place-border: [w81] -> w56
          n21 = in-place-dvr #3(w60) -> (w81:u8[])  [unwired: 1 out]
          n22 = in-place-dvr #3() -> ()  [unwired: 1 in, 2 out]
        }
        n23 = local read "Com UDP"() -> (w50:T5)
        n24 = call "FPS Counter.vi"() -> ("Numeric"=w46:dbl)  [unwired: 11 in]
        "FPS vision" <- w46
        n25 = Build Array("Team", "Side") -> (w52:u16[])
        n26 = Build Array("Id camera\nsup esq", "Id camera\ninf esq", "Id camera\ninf dir", "Id camera\nsup dir") -> (w57:dbl[])
        n27 = in-place {
          in-place-border: [w83] -> w80
          # "Lê da\nreferência(na memória)\ncriada"
          n28 = in-place-dvr #4(w79) -> (w83:T14)  [unwired: 1 out]
          n29 = in-place-dvr #4() -> ()  [unwired: 1 in, 2 out]
        }
        n30 = Build Array("ignore left?", "ignore rigth?") -> (w54:bool[])
        n31 = call "receiveDecodeAndDoKalman.vi"("Vision in"=w55, "cameras array"=w57, "Ignore left/rigth?"=w54, "unsigned byte array"=w56, "Com UDP"=w50, "Estimador"="Estimador", "ball"="ball velocity máx", "team/side"=w52, "ball out"="ball out", "Fps"=w46) -> ("Vision out"=w47:refnum<class "Vision.lvclass">, "Frame and Field Size out"=w53:T19, "error out"=w51:errorcluster)  [unwired: 3 in]
        n32 = in-place {
          in-place-border: [w82] -> w63
          n33 = in-place-dvr #5(w65) -> (w82:refnum<class "Game.lvclass">)  [unwired: 1 out]
          n34 = in-place-dvr #5() -> ()  [unwired: 1 in, 2 out]
        }
        n35 = call "teamAndSide.vi"("Goalie"="Goalie", "team/side"=w52, "error in (no error)"=w51, "Game Status"=w80, "Field State Input"=w53, "Vision in"=w47) -> ("error out"=w75:errorcluster, "IA State"=w49:T24)  [unwired: 3 in, 1 out]
        "AI State" <- w49
        n36 = Unbundle By Name(w49) -> ()  [unwired: 1 out]
        n37 = property class="Game"(reference=w63) -> ("EventsRef"=w62:refnum<class "Events.lvclass">)  [unwired: 1 in, 2 out]
        n38 = Get Date/Time In Seconds() -> (seconds since 1Jan1904=w44:timestamp)
        n39 = feedback-in #6(w44) -> ()
        n40 = feedback #6(w44) -> (w45:timestamp)
        n41 = call "oldVisionToGame.vi"("Defense stretch"="Defense\n stretch", "Team/ Side"=w52, "Defense width"="Defense\n width", "error in (no error)"=w75, "events ref"=w62, "IA State"=w49, "Game in"=w64) -> ("Game out"=w78:refnum<class "Game.lvclass">)  [unwired: 3 in, 1 out]
        n42 = Subtract(x=w44, y=w45) -> (x-y=w43:dbl)
        n43 = local read "tempo udp"() -> (w42:dbl)
        n44 = call "SetVisionFPS.vi"("tempo UDP"=w42, "tempo Vision"=w43, "Vision in"=w47) -> ("milliseconds to wait"=w41:dbl)  [unwired: 6 in, 2 out]
        n45 = Wait (ms)(milliseconds to wait=w41) -> ()  [unwired: 1 out]
      }
      frame #1 {
        n46 = in-place {
          in-place-border: w86 -> [w90]
          n47 = in-place-dvr #7(w87) -> (w91:refnum<class "Game.lvclass">)  [unwired: 1 out]
          n48 = call "BundleAll.vi"("Game in\natualized"=w90, "Game in"=w91) -> ("Game out"=w89:refnum<class "Game.lvclass">)  [unwired: 8 in, 1 out]
          n49 = in-place-dvr #7(w89) -> ()  [unwired: 2 out]
        }
        n50 = in-place {
          in-place-border: w84 -> [w88]
          n51 = in-place-dvr #8(w85) -> ()  [unwired: 2 out]
          n52 = in-place-dvr #8(w88) -> ()  [unwired: 2 out]
        }
      }
    }
  }
  n53 = while {
    tunnel: w4 -> [w98]
    tunnel: w10 -> [w93]
    stop <- FALSE stop-if-true
    # "Get Referee Information"
    n54 = flat-sequence {
      tunnel: w98 -> [w104]
      tunnel: [w100] -> w94
      tunnel: w93 -> [w100]
      tunnel: [w99] -> w92
      tunnel: w94 -> [w107]
      tunnel: w92 -> [w106]
      frame #0 {
        # "Get and decode information about\nde referee commands"
        n55 = call "filterReferee.vi"("Command"="Command", "RefBox UDP RX"="RefBox UDP RX", "Vision in"=w104) -> ("SSL Referee Game Status"=w99:T14, "GUI Game Status"=→"GUI Game Status":T14, "RX"=→"RefBox RX":bool)  [unwired: 4 in, 2 out]
        "SSL Referee Game Status" <- w99
      }
      frame #1 {
        n56 = in-place {
          in-place-border: w106 -> [w108]
          # "Escreve na\nreferência(na memória)\n criada"
          n57 = in-place-dvr #9(w107) -> ()  [unwired: 2 out]
          n58 = in-place-dvr #9(w108) -> ()  [unwired: 2 out]
        }
      }
    }
    n59 = call "FPS Counter.vi"() -> ("Numeric"=→"FPS referee":dbl)  [unwired: 11 in]
    n60 = Wait (ms)(milliseconds to wait=u32 4) -> ()  [unwired: 1 out]
  }
  n61 = while {
    shift-right: [w114] -> _
    shift-left: 0.5 ("New Scale") -> [w121]
    shift-right: [w116] -> _
    shift-left: TRUE ("AutoScale Out") -> [w122]
    tunnel: w4 -> [w120]
    tunnel: w1 -> [w119]
    tunnel: w6 -> [w118]
    stop <- FALSE stop-if-true
    # "Wait necessario\npara 25 FPS"
    # "Draw Field"
    n62 = call "FPS Counter.vi"() -> ("Numeric"=→"FPS Draw Field":dbl)  [unwired: 11 in]
    n63 = feedback #10(0.5 ("New Scale")) -> (w113:dbl)
    n64 = feedback #11(TRUE ("AutoScale Out")) -> (w115:bool)
    n65 = case shown="True" "Draw Field" {
      tunnel: [w123 w134] -> w114
      tunnel: [w124 w133] -> w116
      tunnel: w122 -> [_ w132]
      tunnel: w121 -> [_ w131]
      tunnel: w120 -> [_ w130]
      tunnel: w119 -> [_ w129]
      tunnel: w118 -> [_ w128]
      tunnel: w115 -> [w124 _]
      tunnel: w113 -> [w123 _]
      frame False {
      }
      frame True {
        n66 = flat-sequence {
          tunnel: w132 -> [w143]
          tunnel: w131 -> [w142]
          tunnel: w130 -> [w139]
          tunnel: w129 -> [w138]
          tunnel: w128 -> [w137]
          tunnel: [w145] -> w127
          tunnel: [w144] -> w126
          tunnel: [w135] -> w125
          tunnel: [w157] -> w133
          tunnel: [w158] -> w134
          tunnel: w127 -> [w158]
          tunnel: w126 -> [w157]
          tunnel: w125 -> [w156]
          frame #0 {
            n67 = disable-structure shown="Enabled" {
              disable-tunnel: [w147 1.0 ("Zoom")] -> w141
              frame Enabled {
                n68 = event shown="[0] \"2D Picture\": Mouse Wheel" {
                  selector: _ -> [_ _]
                  dyn-events: _ -> [_ _]
                  timeout: 0 -> [_ _]
                  tunnel: [w148 1.0] -> w147
                  event "2D Picture": Mouse Wheel {
                    n69 = event-data() -> ("Delta"=w152:i32)  [unwired: 1 in]
                    n70 = Greater Than 0?(x=w152) -> (x > 0?=w151:bool)
                    n71 = Select(t=1.2, s=w151, f=0.8) -> (s? t:f=w148:dbl)
                  }
                  event Timeout {
                    n72 = event-data() -> ()  [unwired: 1 in, 3 out]
                  }
                }
              }
              frame Disabled {
              }
            }
            n73 = in-place {
              in-place-border: [w155] -> w136
              n74 = in-place-dvr #12(w137) -> (w155:T19)  [unwired: 1 out]
              n75 = in-place-dvr #12() -> ()  [unwired: 1 in, 2 out]
            }
            n76 = call "drawField.vi"("Vision in"=w139, "AutoScale"=w143, "Game reference"=w138, "Field State Input"=w136, "Scale mm/pixel"=w142, "Draw Targets?"="Draw Targets?", "Zoom"=w141) -> ("AutoScale Out"=w144:bool, "2D Picture"=w135:picture, "Scale Out"=w145:dbl)  [unwired: 4 in, 2 out]
          }
          frame #1 {
            n77 = property on="2D Picture" class="Pict"("Value"=w156) -> ()  [unwired: 2 in, 2 out]
            "2D Picture" <- w156
          }
        }
      }
    }
    n78 = feedback-in #10(w114) -> ()
    n79 = feedback-in #11(w116) -> ()
  }
  n80 = disable-structure shown="Enabled" {
    frame Disabled {
      n81 = while {
        stop <- FALSE stop-if-true
        n82 = event shown="[0] \"2D Picture\": Mouse Wheel" {
          selector: _ -> [_ _]
          dyn-events: _ -> [_ _]
          timeout: 0 -> [_ _]
          tunnel: [w164 1.0] -> w161
          event "2D Picture": Mouse Wheel {
            n83 = event-data() -> ("Delta"=w168:i32)  [unwired: 1 in]
            n84 = Greater Than 0?(x=w168) -> (x > 0?=w167:bool)
            n85 = Select(t=1.2, s=w167, f=0.8) -> (s? t:f=w164:dbl)
          }
          event Timeout {
            n86 = event-data() -> ()  [unwired: 1 in, 3 out]
          }
        }
        "zoom" <- w161
        n87 = call "FPS Counter.vi"() -> ("Numeric"=→"FPS Mouse":dbl)  [unwired: 11 in]
        n88 = Wait (ms)(milliseconds to wait=u32 10) -> ()  [unwired: 1 out]
      }
    }
    frame Enabled {
      n89 = while {
        stop <- FALSE stop-if-true
        # "Wait necessario\npara 25 FPS"
        n90 = call "FPS Counter.vi"() -> ("Numeric"=→"FPS Print Field":dbl)  [unwired: 11 in]
        n91 = Wait (ms)(milliseconds to wait=u32 20) -> ()  [unwired: 1 out]
        n92 = property on="2D Picture" class="Pict" props=["Value"]() -> ()  [unwired: 2 in, 3 out]
      }
    }
  }
  n93 = disable-structure shown="Enabled" {
    disable-tunnel: w1 -> [w173 _]
    frame Enabled {
      n94 = while {
        tunnel: w173 -> [w181]
        stop <- FALSE stop-if-true
        n95 = disable-structure shown="Enabled" {
          frame Disabled {
            n96 = local read "FPS vision"() -> (w187:dbl)
            n97 = Bundle("FPS vision"=w187) -> (w186:cluster{"FPS vision":dbl})  [unwired: 1 in]
            n98 = local read "FPS Navigation"() -> (w184:dbl)
            n99 = local read "FPS Offensive"() -> (w185:dbl)
            n100 = local read "FPS Com"() -> (w183:dbl)
            n101 = Bundle("FPS Navigation"=w184) -> ()  [unwired: 1 in, 1 out]
            n102 = Bundle("FPS Com"=w183) -> ()  [unwired: 1 in, 1 out]
            n103 = Bundle("FPS Offensive"=w185) -> ()  [unwired: 1 in, 1 out]
          }
          frame Enabled {
          }
        }
        n104 = call "FPS Counter.vi"() -> ("Numeric"=→"FPS Graph":dbl)  [unwired: 11 in]
        n105 = in-place {
          in-place-border: [w188] -> w174
          n106 = in-place-dvr #13(w181) -> (w188:refnum<class "Game.lvclass">)  [unwired: 1 out]
          n107 = in-place-dvr #13() -> ()  [unwired: 1 in, 2 out]
        }
        n108 = Wait (ms)(milliseconds to wait=u32 45) -> ()  [unwired: 1 out]
        n109 = case shown="True" "Draw Graphs" {
          tunnel: w174 -> [_ w196]
          tunnel: "id 1" -> [_ w191]
          tunnel: "id 2" -> [_ w190]
          tunnel: "id 3" -> [_ w189]
          frame False {
          }
          frame True {
            n110 = call-dynamic "PlotGraphs.vi"("Game in"=w196, "id 1"=w191, "id 2"=w190, "id 3"=w189) -> ("ball"=→"ball":dbl, "Robot 1"=→"Robot":cluster{"Modulo":dbl, "Modulo":dbl}, "Robot 2"=→"Robot":cluster{"Modulo":dbl, "Modulo":dbl}, "Robot 3"=→"Robot":cluster{"Modulo":dbl, "Modulo":dbl})  [unwired: 6 in, 2 out]
          }
        }
      }
    }
    frame Disabled {
    }
  }
  n111 = while {
    tunnel: w1 -> [w206]
    stop <- FALSE stop-if-true
    # "Event Generator"
    n112 = local read "FPS vision"() -> (w199:dbl)
    n113 = flat-sequence {
      tunnel: w206 -> [w211]
      tunnel: [w208] -> w205
      tunnel: [w207] -> w204
      tunnel: w205 -> [w214]
      tunnel: w204 -> [w213]
      frame #0 {
        n114 = in-place {
          in-place-border: [w212] -> w210
          n115 = in-place-dvr #14(w211) -> (w212:refnum<class "Game.lvclass">)  [unwired: 1 out]
          n116 = in-place-dvr #14() -> (w208:refnum<data-value>)  [unwired: 1 in, 1 out]
        }
        n117 = call-dynamic "Generate_events.vi"("Game in"=w210, "Events in"=refnum<class "Events.lvclass"> refnum) -> ("Events out"=w207:refnum<class "Events.lvclass">)  [unwired: 8 in, 1 out]
      }
      frame #1 {
        n118 = in-place {
          in-place-border: w213 -> [w216]
          n119 = in-place-dvr #15(w214) -> (w217:refnum<class "Game.lvclass">)  [unwired: 1 out]
          n120 = property class="Game"(reference=w217, "EventsRef"=w216) -> (reference out=w215:refnum<class "Game.lvclass">)  [unwired: 1 in, 1 out]
          n121 = in-place-dvr #15(w215) -> ()  [unwired: 2 out]
        }
      }
    }
    n122 = Subtract(x=w199, y=2.0) -> (x-y=w197:dbl)
    n123 = call "FPS Counter.vi"() -> ("Numeric"=→"FPS Events":dbl)  [unwired: 11 in]
    n124 = Divide(x=1000.0, y=w197) -> (x/y=w200:dbl)
    n125 = Wait (ms)(milliseconds to wait=w200) -> ()  [unwired: 1 out]
  }
  n126 = while {
    tunnel: w1 -> [w238]
    stop <- FALSE stop-if-true
    # "Set Parameters"
    n127 = flat-sequence {
      tunnel: w238 -> [w242]
      tunnel: [w242] -> w234
      tunnel: ["Offensive ids"] -> w233
      tunnel: ["Defensive ids"] -> w232
      tunnel: ["zigzag Points"] -> w231
      tunnel: ["TestMode IDS"] -> w230
      tunnel: ["TestMode"] -> w229
      tunnel: ["Tests"] -> w228
      tunnel: ["Test"] -> w227
      tunnel: ["AI Parameters"] -> w226
      tunnel: ["AttakingOurselves"] -> w225
      tunnel: ["Debug"] -> w224
      tunnel: ["ChipKick activated"] -> w223
      tunnel: ["PID gains Vel D"] -> w222
      tunnel: ["PID gains Angle"] -> w221
      tunnel: w234 -> [w265]
      tunnel: w233 -> [w267]
      tunnel: w232 -> [w266]
      tunnel: w231 -> [w264]
      tunnel: w230 -> [w263]
      tunnel: w229 -> [w262]
      tunnel: w228 -> [w261]
      tunnel: w227 -> [w260]
      tunnel: w226 -> [w259]
      tunnel: w225 -> [w258]
      tunnel: w224 -> [w257]
      tunnel: w223 -> [w256]
      tunnel: w222 -> [w255]
      tunnel: w221 -> [w254]
      frame #0 {
      }
      frame #1 {
        n128 = in-place {
          in-place-border: w267 -> [w323]
          in-place-border: w266 -> [w322]
          in-place-border: w264 -> [w271]
          in-place-border: w263 -> [w317]
          in-place-border: w262 -> [w316]
          in-place-border: w261 -> [w315]
          in-place-border: w260 -> [w313]
          in-place-border: w259 -> [w312]
          in-place-border: w258 -> [w279]
          in-place-border: w257 -> [w276]
          in-place-border: w256 -> [w278]
          in-place-border: w255 -> [w274]
          in-place-border: w254 -> [w273]
          n129 = in-place-dvr #16(w265) -> (w324:refnum<class "Game.lvclass">)  [unwired: 1 out]
          n130 = property class="Game"(reference=w324, "Offensive ids"=w323, "Defensive ids"=w322, "Test"=w313, "TestMode IDs"=w317, "TestMode"=w316, "Tests"=w315) -> (reference out=w320:refnum<class "Game.lvclass">, "Parameters.lvclass"=w321:refnum<class "Parameters.lvclass">)  [unwired: 1 in, 1 out]
          n131 = Unbundle By Name(w312) -> ("Area"=w311:enum16{"Circular", "Square"}, "DistanceBehindAttacker"=w310:dbl, "DistanceInFrontOfAttacker"=w309:dbl, "DistanceStop"=w308:dbl, "DistanceToBallOut"=w307:dbl, "DistanceToGoAroundBall"=w306:dbl, "DistanceToGoAroundBallPass"=w305:dbl, "DistanceToKickingAngle"=w280:dbl, "Force++"=w281:dbl, "KickAngle"=w282:dbl, "KickEps"=w283:dbl, "KickForce"=w284:dbl, "KickRange"=w285:dbl, "MaxAcceleration"=w286:dbl, "MaxControlIncrement"=w287:dbl, "MaxDeceleration"=w288:dbl, "MaxOutputAngle"=w289:dbl, "MaxOutputXY"=w290:dbl, "MinDistToKick"=w291:dbl, "PassAngle"=w292:dbl, "Type of Defense"=w293:enum16{"Barreira", "Manmark"}, "Type of Marker"=w294:enum16{"BlockEnemyPass", "BlockOurGoal"}, "AttackerFarback"=w295:dbl, "TouchDistance"=w296:dbl, "TimeoutDistanceInY"=w297:dbl, "TimeoutDistanceInX"=w298:dbl, "TimeoutDistanceBetweenRobots"=w299:dbl, "MaxVelBallToBeginDuelist"=w300:dbl, "DistanceForPossession"=w301:dbl, "DistanceForaStillBall"=w302:dbl, "Defensive Marker"=w303:enum16{"SecondMostDangerous", "MostDangerous"}, "AngularToleranceForPossession"=w304:dbl, "ZigZagAngle"=w277:dbl, "PID gains Vel"=w275:T35, "Number of Offensive"=w272:T36, "Shoot Out?"=w270:bool, "DefenseAvoidArea"=w269:bool, "InvertKick"=w268:dbl[])
          n132 = property class="Parameters.lvclass"(reference=w321, "Area"=w311, "DistanceBehindAttacker"=w310, "DistanceInFrontOfAttacker"=w309, "DistanceStop"=w308, "DistanceToBallOut"=w307, "DistanceToGoAroundBall"=w306, "DistanceToGoAroundBallPass"=w305, "DistanceToKickingAngle"=w280, "Force++"=w281, "KickAngle"=w282, "KickEps"=w283, "KickForce"=w284, "KickRange"=w285, "MaxAcceleration"=w286, "MaxControlIncrement"=w287, "MaxDeceleration"=w288, "MaxOutputAngle"=w289, "MaxOutputXY"=w290, "MinDistToKick"=w291, "PassAngle"=w292, "Type of Defense"=w293, "Type of Marker"=w294, "AttackerFarback"=w295, "TouchDistance"=w296, "TimeoutDistanceInY"=w297, "TimeoutDistanceInX"=w298, "TimeoutDistanceBetweenRobots"=w299, "MaxVelBallToBeginDuelist"=w300, "DistanceForPossession"=w301, "DistanceForaStillBall"=w302, "Defensive Marker"=w303, "AngularToleranceForPossession"=w304, "zigzag Points"=w271, "AttakingOurselves"=w279, "Debug"=w276, "ChipKick activated"=w278, "Angle"=w277, "PID gains Vel"=w275, "PID gains Vel_desired"=w274, "PID gains Angle"=w273, "Number of Offesnive"=w272, "Shoot Out_"=w270, "DefenseAvoidArea"=w269, "InvertKick"=w268) -> (reference out=w318:refnum<class "Parameters.lvclass">, error out=→"error out":errorcluster)  [unwired: 1 in]
          n133 = property class="Game"(reference=w320, "Parameters.lvclass"=w318) -> (reference out=w319:refnum<class "Game.lvclass">)  [unwired: 1 in, 1 out]
          n134 = in-place-dvr #16(w319) -> ()  [unwired: 2 out]
        }
      }
    }
    n135 = local read "FPS vision"() -> (w220:dbl)
    n136 = call "FPS Counter.vi"() -> ("Numeric"=→"FPS SetParameters":dbl)  [unwired: 11 in]
    n137 = Subtract(x=w220, y=2.0) -> (x-y=w218:dbl)
    n138 = Divide(x=1000.0, y=w218) -> (x/y=w235:dbl)
    n139 = Wait (ms)(milliseconds to wait=w235) -> ()  [unwired: 1 out]
  }
  n140 = while {
    tunnel: w1 -> [w334]
    stop <- FALSE stop-if-true
    # "Offensive"
    n141 = local read "FPS vision"() -> (w325:dbl)
    n142 = flat-sequence {
      tunnel: w334 -> [w353]
      tunnel: [w350] -> w331
      tunnel: [w349] -> w330
      tunnel: [w348] -> w329
      tunnel: w326 -> [w345]
      tunnel: w325 -> [w342]
      tunnel: w331 -> [w357]
      tunnel: w330 -> [w356]
      tunnel: w329 -> [w355]
      frame #0 {
        w341 = 30.0
        # "Pass unique line"
        n143 = in-place {
          in-place-border: [w354] -> w346
          n144 = in-place-dvr #17(w353) -> (w354:refnum<class "Game.lvclass">)  [unwired: 1 out]
          n145 = in-place-dvr #17() -> (w348:refnum<data-value>)  [unwired: 1 in, 1 out]
        }
        n146 = call-dynamic "chooseOffensivePlay.vi"("Game in"=w346) -> ("error out"=w352:errorcluster, "Game out"=w351:refnum<class "Game.lvclass">)  [unwired: 9 in]
        n147 = call-dynamic "pickOffensiveRobots.vi"("error in (no error)"=w352, "Game in"=w351) -> ("error out"=w337:errorcluster, "Game out"=w339:refnum<class "Game.lvclass">)  [unwired: 8 in]
        n148 = call-dynamic "executeOffensivePlay.vi"("error in (no error)"=w337, "Game in"=w339) -> ("error out"=w336:errorcluster, "Game out"=w338:refnum<class "Game.lvclass">)  [unwired: 8 in]
        n149 = Greater Or Equal?(x=w342, y=w341) -> (x >= y?=w343:bool)
        n150 = Less Or Equal?(x=w345, y=w341) -> (x <= y?=w344:bool)
        n151 = And(x=w343, y=w344) -> (x .and. y?=w340:bool)
        n152 = call-dynamic "pathPlanningOffensive.vi"("error in (no error)"=w336, "Line?"=w340, "Game in"=w338) -> ("Game out"=w347:refnum<class "Game.lvclass">)  [unwired: 7 in, 1 out]
        n153 = property class="Game"(reference=w347) -> ("OffensiveTeam"=w350:refnum<class "Ally.lvclass">, "Playbook"=w349:refnum<class "Playbook.lvclass">)  [unwired: 1 in, 2 out]
      }
      frame #1 {
        n154 = in-place {
          in-place-border: w357 -> [w361]
          in-place-border: w356 -> [w360]
          n155 = in-place-dvr #18(w355) -> (w358:refnum<class "Game.lvclass">)  [unwired: 1 out]
          n156 = property class="Game"(reference=w358, "OffensiveTeam"=w361, "Playbook"=w360) -> (reference out=w359:refnum<class "Game.lvclass">)  [unwired: 1 in, 1 out]
          n157 = in-place-dvr #18(w359) -> ()  [unwired: 2 out]
        }
      }
    }
    n158 = Subtract(x=w325, y=2.0) -> (x-y=w328:dbl)
    n159 = Divide(x=1000.0, y=w328) -> (x/y=w332:dbl)
    n160 = Wait (ms)(milliseconds to wait=w332) -> ()  [unwired: 1 out]
    n161 = call "FPS Counter.vi"() -> ("Numeric"=w326:dbl)  [unwired: 11 in]
    "FPS Offensive" <- w326
  }
  n162 = while {
    tunnel: w1 -> [w371]
    stop <- FALSE stop-if-true
    # "Keeper"
    n163 = local read "FPS vision 2"() -> (w362:dbl)
    n164 = flat-sequence {
      tunnel: w371 -> [w389]
      tunnel: [w388] -> w368
      tunnel: [w387] -> w367
      tunnel: [w386] -> w366
      tunnel: w363 -> [w385]
      tunnel: w362 -> [w382]
      tunnel: w368 -> [w393]
      tunnel: w367 -> [w392]
      tunnel: w366 -> [w391]
      frame #0 {
        w381 = 30.0
        # "Pass unique line"
        n165 = in-place {
          in-place-border: [w390] -> w380
          n166 = in-place-dvr #19(w389) -> (w390:refnum<class "Game.lvclass">)  [unwired: 1 out]
          n167 = in-place-dvr #19() -> (w386:refnum<data-value>)  [unwired: 1 in, 1 out]
        }
        n168 = call "chooseKeeperPlay.vi"("Game in"=w380) -> ("error out"=w378:errorcluster, "Game out"=w379:refnum<class "Game.lvclass">)  [unwired: 9 in]
        n169 = call-dynamic "pickKeeperRobots.vi"("error in (no error)"=w378, "Game in"=w379) -> ("error out"=w376:errorcluster, "Game out"=w377:refnum<class "Game.lvclass">)  [unwired: 8 in]
        n170 = call-dynamic "executeKeeperPlay.vi"("error in (no error)"=w376, "Game in"=w377) -> ("error out"=w374:errorcluster, "Game out"=w375:refnum<class "Game.lvclass">)  [unwired: 8 in]
        n171 = Greater Or Equal?(x=w382, y=w381) -> (x >= y?=w383:bool)
        n172 = Less Or Equal?(x=w385, y=w381) -> (x <= y?=w384:bool)
        n173 = And(x=w383, y=w384) -> ()  [unwired: 1 out]
        n174 = call-dynamic "pathPlanningKeeper.vi"("error in (no error)"=w374, "Game in"=w375) -> ("Game out"=w373:refnum<class "Game.lvclass">)  [unwired: 8 in, 1 out]
        n175 = property class="Game"(reference=w373) -> ("KeeperTeam"=w388:refnum<class "Ally.lvclass">, "Playbook"=w387:refnum<class "Playbook.lvclass">)  [unwired: 1 in, 2 out]
      }
      frame #1 {
        n176 = in-place {
          in-place-border: w393 -> [w397]
          in-place-border: w392 -> [w396]
          n177 = in-place-dvr #20(w391) -> (w394:refnum<class "Game.lvclass">)  [unwired: 1 out]
          n178 = property class="Game"(reference=w394, "KeeperTeam"=w397, "Playbook"=w396) -> (reference out=w395:refnum<class "Game.lvclass">)  [unwired: 1 in, 1 out]
          n179 = in-place-dvr #20(w395) -> ()  [unwired: 2 out]
        }
      }
    }
    n180 = Subtract(x=w362, y=2.0) -> (x-y=w365:dbl)
    n181 = Divide(x=1000.0, y=w365) -> (x/y=w369:dbl)
    n182 = Wait (ms)(milliseconds to wait=w369) -> ()  [unwired: 1 out]
    n183 = call "FPS Counter.vi"() -> ("Numeric"=w363:dbl)  [unwired: 11 in]
    "FPS Offensive 2" <- w363
  }
  n184 = while {
    tunnel: w1 -> [w401]
    stop <- FALSE stop-if-true
    # "Navigation"
    n185 = flat-sequence {
      tunnel: [w422] -> w405
      tunnel: w401 -> [w419]
      tunnel: [w409] -> w400
      tunnel: [w407] -> w399
      tunnel: [w436] -> _
      tunnel: w405 -> [w436]
      tunnel: w400 -> [w435]
      tunnel: w399 -> [w434]
      frame #0 {
        n186 = in-place {
          in-place-border: [w433] -> w423
          n187 = in-place-dvr #21(w419) -> (w433:refnum<class "Game.lvclass">)  [unwired: 1 out]
          n188 = in-place-dvr #21() -> (w422:refnum<data-value>)  [unwired: 1 in, 1 out]
        }
        n189 = call-dynamic "NavigationOffensive.vi"("Game in"=w423) -> ("Game out"=w421:refnum<class "Game.lvclass">)  [unwired: 9 in, 1 out]
        n190 = call-dynamic "NavigationDefensive.vi"("Game in"=w423) -> ("Game out"=w420:refnum<class "Game.lvclass">)  [unwired: 9 in, 1 out]
        n191 = call-dynamic "NavigationKeeper.vi"("Game in"=w423) -> ("Game out"=w408:refnum<class "Game.lvclass">)  [unwired: 9 in, 1 out]
        n192 = property class="Game"(reference=w421) -> ("OffensiveTeam"=w411:refnum<class "Ally.lvclass">)  [unwired: 1 in, 2 out]
        n193 = property class="Game"(reference=w420) -> ("DefensiveTeam"=w410:refnum<class "Ally.lvclass">)  [unwired: 1 in, 2 out]
        n194 = property class="Game"(reference=w408) -> ("AllyRef"=w407:refnum<class "Ally.lvclass">)  [unwired: 1 in, 2 out]
        n195 = property class="Game"(reference=w408) -> ("KeeperTeam"=w412:refnum<class "Ally.lvclass">)  [unwired: 1 in, 2 out]
        n196 = property class="Ally"(reference=w410) -> ("RobotRef"=w413:refnum<class "Robot.lvclass">[])  [unwired: 1 in, 2 out]
        n197 = property class="Ally"(reference=w412) -> ("RobotRef"=w418:refnum<class "Robot.lvclass">[])  [unwired: 1 in, 2 out]
        n198 = property class="Ally"(reference=w411) -> ("RobotRef"=w415:refnum<class "Robot.lvclass">[])  [unwired: 1 in, 2 out]
        n199 = for {
          tunnel: w418 -> [w432] mode=indexing
          shift-right: [w430] -> w416
          shift-left: refnum<class "Robot.lvclass">[] [] -> [w431]
          n200 = Insert Into Array(array=w431, new element=w432) -> (w430:refnum<class "Robot.lvclass">[])  [unwired: 1 in]
        }
        n201 = for {
          tunnel: w415 -> [w429] mode=indexing
          shift-right: [w427] -> w414
          shift-left: w416 -> [w428]
          n202 = Insert Into Array(array=w428, new element=w429) -> (w427:refnum<class "Robot.lvclass">[])  [unwired: 1 in]
        }
        n203 = for {
          tunnel: w413 -> [w426] mode=indexing
          shift-right: [w424] -> w409
          shift-left: w414 -> [w425]
          n204 = Insert Into Array(array=w425, new element=w426) -> (w424:refnum<class "Robot.lvclass">[])  [unwired: 1 in]
        }
      }
      frame #1 {
        n205 = in-place {
          in-place-border: w435 -> [w438]
          in-place-border: w434 -> [w437]
          n206 = in-place-dvr #22(w436) -> (w440:refnum<class "Game.lvclass">)  [unwired: 1 out]
          n207 = property class="Ally"(reference=w437, "RobotRef"=w438) -> (reference out=w439:refnum<class "Ally.lvclass">)  [unwired: 1 in, 1 out]
          n208 = property class="Game"(reference=w440, "NavigationTeam"=w439) -> (reference out=w441:refnum<class "Game.lvclass">)  [unwired: 1 in, 1 out]
          n209 = in-place-dvr #22(w441) -> ()  [unwired: 2 out]
        }
      }
    }
    n210 = call "FPS Counter.vi"() -> ("Numeric"=→"FPS Navigation":dbl)  [unwired: 11 in]
    n211 = Divide(x=1000.0, y=30.0) -> (x/y=w404:dbl)
    n212 = Wait (ms)(milliseconds to wait=w404) -> ()  [unwired: 1 out]
  }
  n213 = while {
    tunnel: w1 -> [w472]
    stop <- FALSE stop-if-true
    n214 = local read "FPS vision"() -> (w450:dbl)
    n215 = Subtract(x=w450, y=5.0) -> (x-y=w447:dbl)
    n216 = in-place {
      in-place-border: [w507] -> w445
      n217 = in-place-dvr #23(w472) -> (w507:refnum<class "Game.lvclass">)  [unwired: 1 out]
      n218 = in-place-dvr #23() -> (w467:refnum<data-value>)  [unwired: 1 in, 1 out]
    }
    n219 = disable-structure shown="Disabled" {
      disable-tunnel: w445 -> [w487 _]
      frame Disabled {
        w476 = refnum<class "Utilities.lvclass"> refnum ("Utilities in")
        n220 = property class="Game"(reference=w487) -> ("NavigationTeam"=w486:refnum<class "Ally.lvclass">)  [unwired: 1 in, 2 out]
        n221 = property class="Ally"(reference=w486) -> ("RobotRef"=w485:refnum<class "Robot.lvclass">[])  [unwired: 1 in, 2 out]
        n222 = Index Array(array=w485) -> (element=w484:refnum<class "Robot.lvclass">)  [unwired: 1 in]
        n223 = property class="Robot"(reference=w484) -> ("v_norm"=w480:dbl, "v_tang"=w479:dbl, "est_v_norm"=w475:dbl, "est_v_tang"=w474:dbl)  [unwired: 1 in, 2 out]
        n224 = Build Array(w480, w479) -> (w483:dbl[])
        n225 = call-dynamic "Module.vi"("2D vector"=w483, "Utilities in"=w476) -> ("Modulo"=w482:dbl)  [unwired: 7 in, 2 out]
        n226 = Build Array(w475, w474) -> (w477:dbl[])
        n227 = Bundle("v_norm"=w480, "v_tang"=w479, "Modulo"=w482) -> (→"Vel cmd":T3)  [unwired: 1 in]
        n228 = call-dynamic "Module.vi"("2D vector"=w477, "Utilities in"=w476) -> ("Modulo"=w478:dbl)  [unwired: 7 in, 2 out]
        n229 = Bundle("est_v_norm"=w475, "est_v_tang"=w474, "Modulo"=w478) -> (→"Vel estimativa":T37)  [unwired: 1 in]
      }
      frame Enabled {
      }
    }
    n230 = Divide(x=1000.0, y=w447) -> (x/y=w451:dbl)
    n231 = Wait (ms)(milliseconds to wait=w451) -> ()  [unwired: 1 out]
    n232 = call-dynamic "communicate.vi"("Communication in"="Communication in", "grSIM replacement"="grSIM replacement", "replace active"="replace active", "Game"=w445, "Com UDP"="Com UDP", "Com Serial"="Com Serial", "Com SOS"="Com SOS") -> ("Comm TX FPS"=→"FPS Com":dbl, "AllyRef"=w468:refnum<class "Ally.lvclass">)  [unwired: 5 in, 2 out]
    n233 = disable-structure shown="Disabled" {
      disable-tunnel: w468 -> [w489 _]
      disable-tunnel: w467 -> [w488 _]
      frame Disabled {
        n234 = in-place {
          in-place-border: w489 -> [w490]
          n235 = in-place-dvr #24(w488) -> (w491:refnum<class "Game.lvclass">)  [unwired: 1 out]
          n236 = property class="Game"(reference=w491, "AllyRef"=w490) -> ()  [unwired: 1 in, 2 out]
          n237 = in-place-dvr #24() -> ()  [unwired: 1 in, 2 out]
        }
      }
      frame Enabled {
      }
    }
    n238 = property class="Game"(reference=w467) -> ("Referee"=w457:refnum<class "Referee.lvclass">, "KeeperTeam"=w466:refnum<class "Ally.lvclass">, "OffensiveTeam"=w465:refnum<class "Ally.lvclass">, "DefensiveTeam"=w464:refnum<class "Ally.lvclass">)  [unwired: 1 in, 2 out]
    n239 = property class="Ally"(reference=w464) -> ("RobotRef"=w461:refnum<class "Robot.lvclass">[], "DefensivePlay"=→"DefensivePlay":T13)  [unwired: 1 in, 2 out]
    n240 = property class="Ally"(reference=w465) -> ("RobotRef"=w462:refnum<class "Robot.lvclass">[], "OffensivePlay"=→"OffensivePlay":T10)  [unwired: 1 in, 2 out]
    n241 = property class="Ally"(reference=w466) -> ("RobotRef"=w463:refnum<class "Robot.lvclass">[], "KeeperPlay"=→"KeeperPlay":T9)  [unwired: 1 in, 2 out]
    n242 = property class="Referee"(reference=w457) -> ("command_interpreted"=→"command_interpreted":T15)  [unwired: 1 in, 2 out]
    n243 = for {
      tunnel: w462 -> [w501] mode=indexing
      tunnel: [w498] -> w454 mode=indexing
      n244 = property class="Robot"(reference=w501) -> ("id"=w500:i32, "role"=w499:T11, "tactic"=w497:T12)  [unwired: 1 in, 2 out]
      n245 = Bundle("id"=w500, "role"=w499, "tactic"=w497) -> (w498:cluster{"id":i32, "role":T11, "tactic":T12})  [unwired: 1 in]
    }
    "Offensive Team" <- w454
    n246 = for {
      tunnel: w463 -> [w506] mode=indexing
      tunnel: [w503] -> w455 mode=indexing
      n247 = property class="Robot"(reference=w506) -> ("id"=w505:i32, "role"=w504:T11, "tactic"=w502:T12)  [unwired: 1 in, 2 out]
      n248 = Bundle("id"=w505, "role"=w504, "tactic"=w502) -> (w503:cluster{"id":i32, "role":T11, "tactic":T12})  [unwired: 1 in]
    }
    "Keeper Team" <- w455
    n249 = for {
      tunnel: w461 -> [w496] mode=indexing
      tunnel: [w493] -> w453 mode=indexing
      n250 = property class="Robot"(reference=w496) -> ("id"=w495:i32, "role"=w494:T11, "tactic"=w492:T12)  [unwired: 1 in, 2 out]
      n251 = Bundle("id"=w495, "role"=w494, "tactic"=w492) -> (w493:cluster{"id":i32, "role":T11, "tactic":T12})  [unwired: 1 in]
    }
    "Defensive Team" <- w453
  }
